vi "SaccadeAnalyser - Calc Fick from Rotation Vector.vi"(2 "Sample Rate (Hz)":dbl=500.0, 3 "Rotation Vectors (XYZ)":dbl[][](array[numeric])) -> (0 "Velocity RALP, LARP, Z (deg/s)":dbl[][](array[numeric]), 1 "Angles Roll, Pitch, Yaw, RALP, LARP (deg)":dbl[][](array[numeric]))   [LabVIEW 2016]
uses:
  <userlib>/Maths/3D Rotation/Conversion/Convert Euler Angles To Quaternion _one.vi
  <userlib>/Maths/3D Rotation/Conversion/Convert Rotation Vector To Quaternion _one.vi
  <userlib>/Maths/3D Rotation/Conversion/Convert Quaternion To Euler Angles _many.vi
  <vilib>/Analysis/NI_AALPro.lvlib
panel:
  # "Reproduced from: Cremer et al, 1998, Semicircular canal plane head impulses detect\nabsent function of individual semicircular canals\n\nhttps://academic.oup.com/brain/article/121/4/699/260859\n\nhttps://doi.org/10.1093/brain/121.4.699"
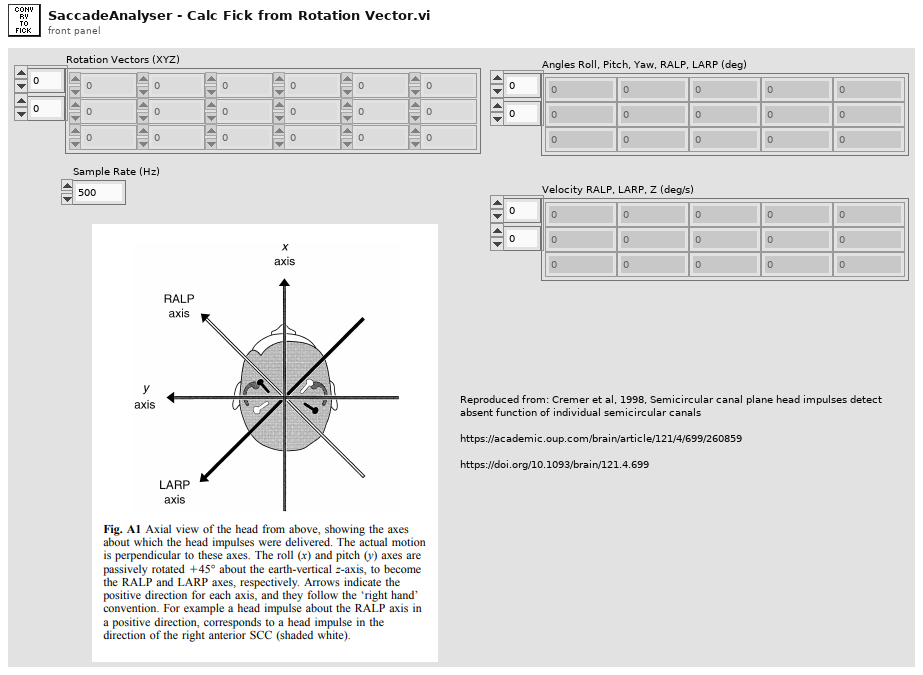
[diagram p1: front panel]
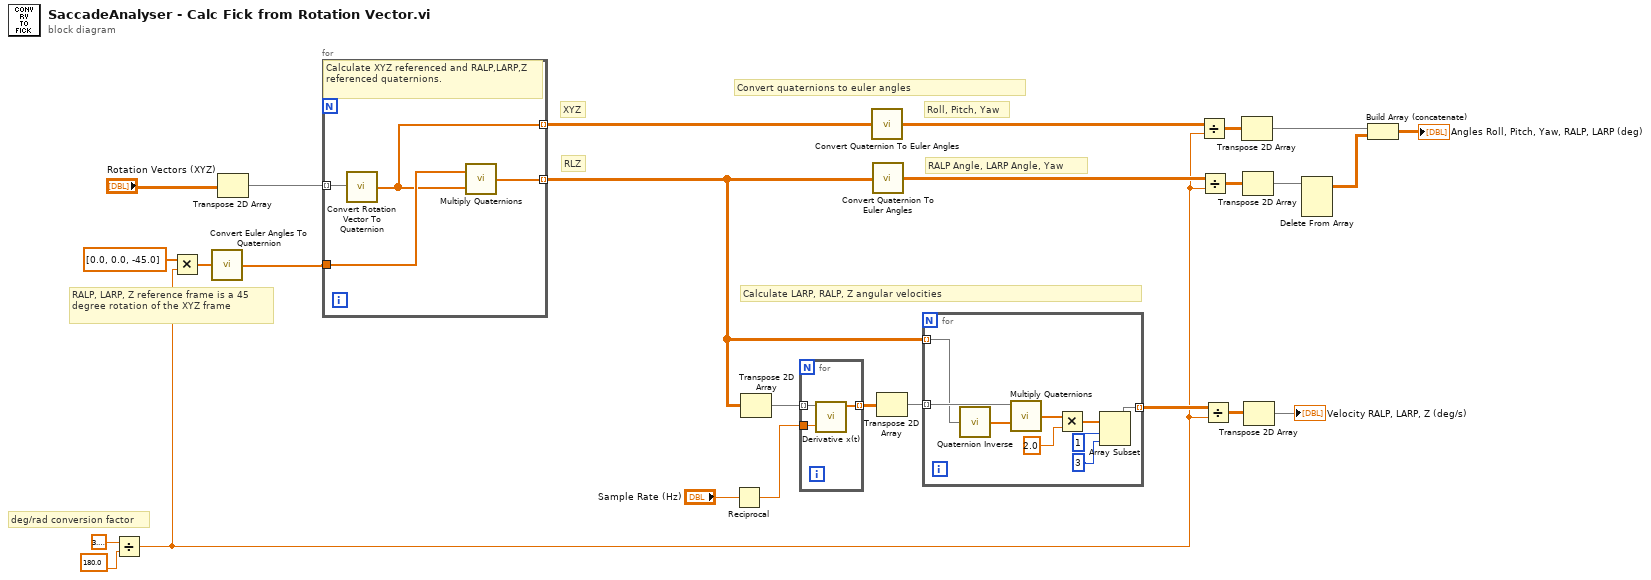
[diagram p0: block diagram]
diagram:
  # "RALP Angle, LARP Angle, Yaw"
  # "Roll, Pitch, Yaw"
  # "RALP, LARP, Z reference frame is a 45 degree rotation of the XYZ frame"
  # "deg/rad conversion factor"
  # "RLZ"
  # "XYZ"
  # "Convert quaternions to euler angles"
  # "Calculate LARP, RALP, Z angular velocities"
  n1 = Divide(x=3.141592653589793, y=180.0) -> (x/y=w6:dbl)
  n2 = Multiply(x=dbl[] [0.0, 0.0, -45.0] ("RPY (rad)"), y=w6) -> (x*y=w25:dbl[])
  n3 = call-poly <userlib>:"Convert Euler Angles To Quaternion.vi"("RPY (rad)"=w25) -> ("Q"=w20:dbl[])
  n4 = Transpose 2D Array(2D array="Rotation Vectors (XYZ)") -> (transposed array=w26:dbl[][])
  n5 = for {
    tunnel: w26 -> [w28] mode=indexing
    tunnel: w20 -> [w30]
    tunnel: [w29] -> w8 mode=indexing
    tunnel: [w27] -> w9 mode=indexing
    # "Calculate XYZ referenced and RALP,LARP,Z referenced quaternions."
    n6 = call-poly <userlib>:"Convert Rotation Vector To Quaternion.vi"("RV"=w28) -> ("Q"=w27:dbl[])
    n7 = call <userlib>:"Multiply Quaternions.vi"("Q2"=w27, "Q1"=w30) -> ("Q"=w29:dbl[])
  }
  n8 = Reciprocal(x="Sample Rate (Hz)") -> (1/x=w13:dbl)
  n9 = Transpose 2D Array(2D array=w8) -> (transposed array=w15:dbl[][])
  n10 = for {
    tunnel: w15 -> [w33] mode=indexing
    tunnel: [w32] -> w12 mode=indexing
    tunnel: w13 -> [w31]
    n11 = call <vilib>:"Derivative x(t).vi"("dt"=w31, "X"=w33) -> ("dX/dt"=w32:dbl[])  [unwired: 8 in, 1 out]
  }
  n12 = call-poly <userlib>:"Convert Quaternion To Euler Angles.vi"("Q"=w9) -> ("RPY (rad)"=w7:dbl[][])
  n13 = call-poly <userlib>:"Convert Quaternion To Euler Angles.vi"("Q"=w8) -> ("RPY (rad)"=w16:dbl[][])
  n14 = Transpose 2D Array(2D array=w12) -> (transposed array=w11:dbl[][])
  n15 = for {
    tunnel: w11 -> [w42] mode=indexing
    tunnel: w8 -> [w40] mode=indexing
    tunnel: [w34] -> w10 mode=indexing
    # "Calc angular velocity by quaternions (americo thesis)"
    n16 = call <userlib>:"Quaternion Inverse.vi"("Q"=w40) -> ("Q Inverse"=w41:dbl[])
    n17 = call <userlib>:"Multiply Quaternions.vi"("Q2"=w41, "Q1"=w42) -> ("Q"=w39:dbl[])
    n18 = Multiply(x=w39, y=2.0) -> (x*y=w37:dbl[])
    n19 = Array Subset(array=w37, index=1, length=3) -> (w34:dbl[])
  }
  n20 = Divide(x=w7, y=w6) -> (x/y=w5:dbl[][])
  n21 = Divide(x=w16, y=w6) -> (x/y=w21:dbl[][])
  n22 = Divide(x=w10, y=w6) -> (x/y=w17:dbl[][])
  n23 = Transpose 2D Array(2D array=w5) -> (transposed array=w3:dbl[][])
  n24 = Transpose 2D Array(2D array=w21) -> (transposed array=w4:dbl[][])
  n25 = Transpose 2D Array(2D array=w17) -> (transposed array=→"Velocity RALP, LARP, Z (deg/s)":dbl[][])
  n26 = Delete From Array(array=w4) -> (array with subset deleted=w2:dbl[][])  [unwired: 3 in, 1 out]
  n27 = Build Array (concatenate)(w3, w2) -> (→"Angles Roll, Pitch, Yaw, RALP, LARP (deg)":dbl[][])
